vi "CAN_ID.vi"() -> ()   [LabVIEW 2019]
panel:
  in  "CAN_ID":T1
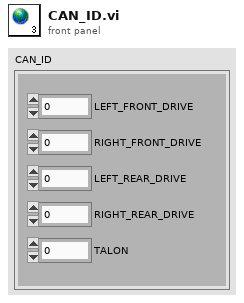
[diagram p1: front panel]
types:
  T1 = cluster{"LEFT_FRONT_DRIVE":u8, "LEFT_REAR_DRIVE":u8, "RIGHT_FRONT_DRIVE":u8, "RIGHT_REAR_DRIVE":u8, "TALON":u8}
diagram:
